vi "HTTP Info.vi"() -> ()   [LabVIEW 2020, in "VectoScratch.lvlib"]
uses:
  VectoScratch.lvlib
  Vecto/Vecto Info.ctl
  Vecto/Connection Info.ctl
  Vecto/Connection Type.ctl
  Vecto/proto/Discovery/Data.ctl
  Vecto/proto/Service/Data.ctl
  Vecto/proto/ServiceType/Enumeration.ctl
  Vecto/Node/Node Info.ctl
  Vecto/Discovery Info.ctl
  Vecto/VectoService/VectoService.lvclass
  C:/dev/lv20CE/lv-vecto/Vecto/Service/Service.lvclass
  Vecto/DiscoveryService/DiscoveryService.lvclass
  Vecto/Node/Node.lvclass
  Vecto/Vecto/Vecto.lvclass
  Vecto/Vecto.lvlib
  Vecto/proto/ServiceType/ServiceType.lvlib
  Vecto/proto/Service/Service.lvlib
  Vecto/proto/Discovery/Discovery.lvlib
panel:
  in  "ID":u32=1
  in  "Start":bool
  out "Discovery":T1[](array[typedef]) {"ip" format="%.0x"}
  in  "Discovery Address":string="230.0.0.50"
  in  "Discovery Port":u16=36986
  out "error out":errorcluster
  out "Vecto Info":T4
  in  "stop":bool
  in  "Node Name":string="Alpha"
  in  "HTTP Port":u16=36987
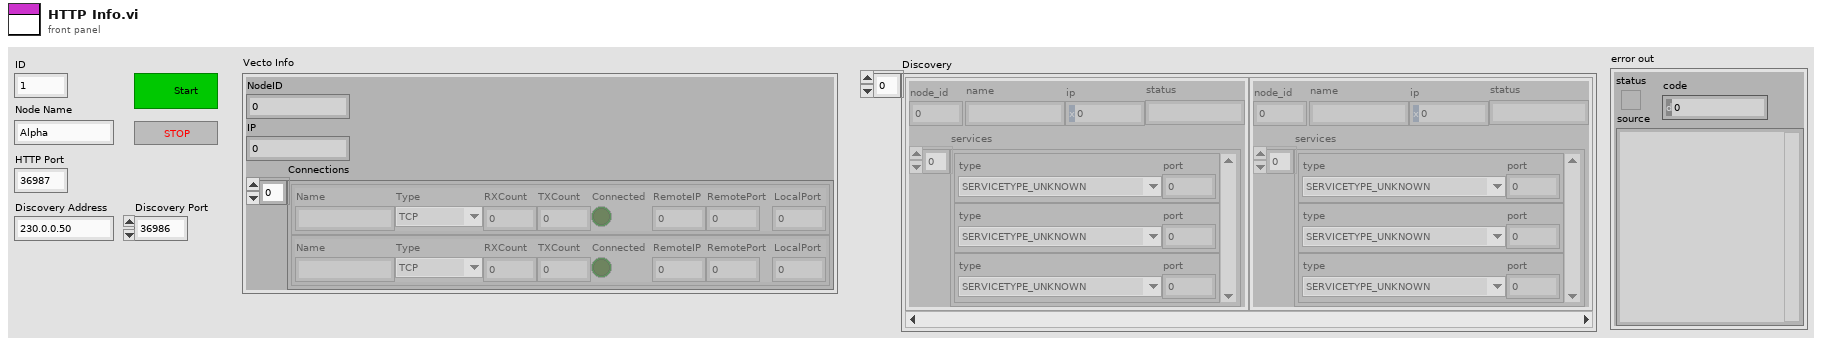
[diagram p1: front panel]
types:
  T1 = typedef "Discovery.lvlib/Data.ctl" = cluster{"node_id":u32, "name":string, "ip":u32, "status":string, "services":T2[]}
  T2 = typedef "Service.lvlib/Data.ctl" = cluster{"type":T3, "port":i32}
  T3 = typedef "ServiceType.lvlib/Enumeration.ctl" = enum16{"SERVICETYPE_UNKNOWN", "SERVICETYPE_TCPSERVER", "SERVICETYPE_HTTPSERVER"}
  T4 = typedef "Vecto.lvlib/Vecto Info.ctl" = cluster{"NodeID":i32, "IP":u32, "Connections":T5[]}
  T5 = typedef "Vecto.lvlib/Connection Info.ctl" = cluster{"Name":string, "Type":T6, "RXCount":i32, "TXCount":i32, "Connected":bool, "RemoteIP":u32, "RemotePort":u16, "LocalPort":u16}
  T6 = typedef "Vecto.lvlib/Connection Type.ctl" = enum16{"TCP", "Telemetry", "Discovery", "HTTP"}
  T7 = typedef "Vecto.lvlib/Discovery Info.ctl" = cluster{"Address":string, "Port":u16, "Interval S":dbl}
  T8 = typedef "Vecto.lvlib/Node.lvclass/Node Info.ctl" = cluster{"HTTP Port":u16, "Bind Address":string}
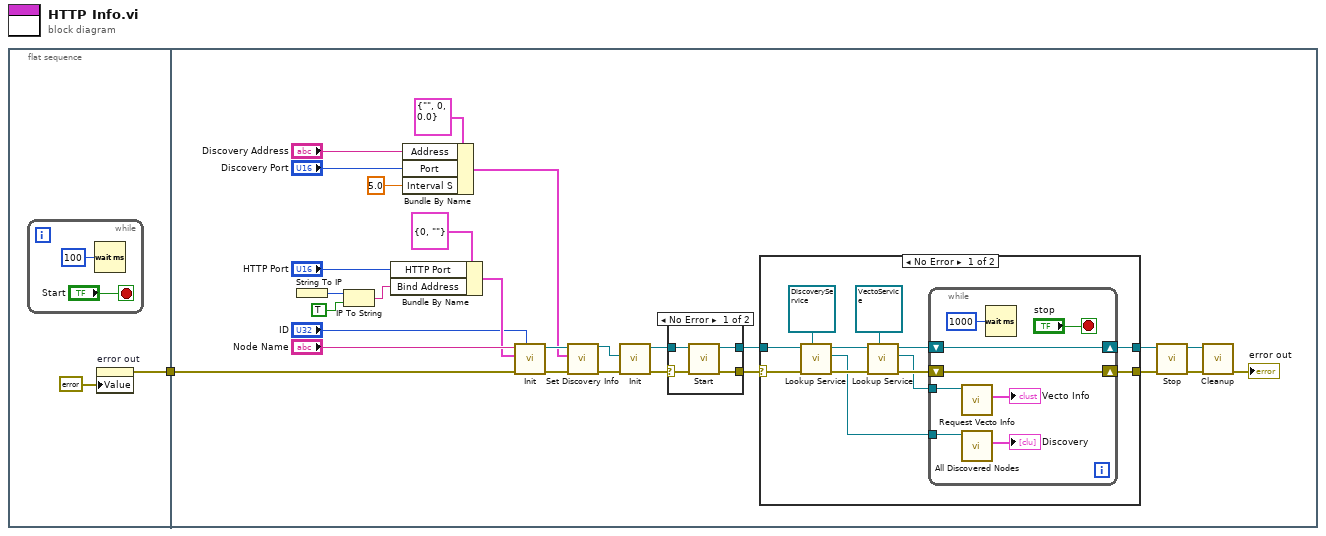
[diagram p0: block diagram]
diagram:
  n1 = flat-sequence {
    tunnel: [w2] -> w1
    tunnel: w1 -> [w7]
    frame #0 {
      n2 = while {
        stop <- "Start" stop-if-true
        n3 = Wait (ms)(milliseconds to wait=u32 100) -> ()  [unwired: 1 out]
      }
      n4 = property on="error out" class="Clust (strict)"("Value"=errorcluster {"status"=FALSE, "code"=0, "source"=""} ("error constant")) -> (error out=w2:errorcluster)  [unwired: 2 in, 1 out]
    }
    frame #1 {
      n5 = String To IP() -> (0:w17:u32)  [unwired: 1 in]
      n6 = IP To String(1:TRUE ("dot notation? (F)"), 2:w17) -> (0:w18:string)
      n7 = Bundle By Name(cluster=T8 {"HTTP Port"=0, "Bind Address"=""} ("Node Info"), "HTTP Port"="HTTP Port", "Bind Address"=w18) -> (w8:T8)
      n8 = Bundle By Name(cluster=T7 {"Address"="", "Port"=0, "Interval S"=0.0} ("Discovery Info"), "Address"="Discovery Address", "Port"="Discovery Port", "Interval S"=5.0) -> (w12:T7)
      n9 = call "Init.vi"("ID"="ID", "error in (no error)"=w7, "Node Info"=w8, "Name"="Node Name") -> ("error out"=w29:errorcluster, "Node out"=w15:refnum<class "Node.lvclass">)  [unwired: 6 in]
      n10 = call "Set Discovery Info.vi"("error in (no error)"=w29, "Discovery Info"=w12, "Node in"=w15) -> ("error out"=w16:errorcluster, "Node out"=w14:refnum<class "Node.lvclass">)  [unwired: 7 in]
      n11 = call "Init.vi"("error in (no error)"=w16, "Node"=w14) -> ("error out"=w28:errorcluster, "Vecto out"=w27:refnum<class "Vecto.lvclass">)  [unwired: 8 in]
      n12 = case shown="No Error" w28 {
        selector: w28 -> [w36 w38]
        tunnel: w27 -> [w35 w37]
        tunnel: [w34 w38] -> w26
        tunnel: [w33 w37] -> w23
        frame No Error {
          n13 = call "Start.vi"("error in (no error)"=w36, "Vecto in"=w35) -> ("error out"=w34:errorcluster, "Vecto out"=w33:refnum<class "Vecto.lvclass">)  [unwired: 8 in]
        }
        frame Error {
        }
      }
      n14 = case shown="No Error" w26 {
        selector: w26 -> [w43 w60]
        tunnel: [w50 w59] -> w25
        tunnel: [w49 w60] -> w24
        tunnel: w23 -> [w44 w59]
        frame No Error {
          n15 = call "Lookup Service.vi"("Service Type / ID"=refnum<class "DiscoveryService.lvclass"> refnum ("Vecto.lvlib:DiscoveryService.lvclass"), "error in (no error)"=w43, "Vecto in"=w44) -> ("error out"=w42:errorcluster, "Service"=w39:refnum<class "DiscoveryService.lvclass">, "Vecto out"=w41:refnum<class "Vecto.lvclass">)  [unwired: 6 in]
          n16 = call "Lookup Service.vi"("Service Type / ID"=refnum<class "VectoService.lvclass"> refnum ("Vecto.lvlib:VectoService.lvclass"), "error in (no error)"=w42, "Vecto in"=w41) -> ("error out"=w48:errorcluster, "Service"=w45:refnum<class "VectoService.lvclass">, "Vecto out"=w47:refnum<class "Vecto.lvclass">)  [unwired: 6 in]
          n17 = while {
            shift-right: [w56] -> w49
            shift-left: w48 -> [w56]
            shift-right: [w57] -> w50
            shift-left: w47 -> [w57]
            tunnel: w45 -> [w54]
            tunnel: w39 -> [w52]
            stop <- "stop" stop-if-true
            n18 = call "Request Vecto Info.vi"("VectoService in"=w54) -> ("Vecto Info"=→"Vecto Info":T4)  [unwired: 8 in, 2 out]
            n19 = call "All Discovered Nodes.vi"("DiscoveryService in"=w52) -> ("Nodes"=→"Discovery":T1[])  [unwired: 8 in, 2 out]
            n20 = Wait (ms)(milliseconds to wait=u32 1000) -> ()  [unwired: 1 out]
          }
        }
        frame Error {
        }
      }
      n21 = call "Stop.vi"("error in (no error)"=w24, "Vecto in"=w25) -> ("error out"=w22:errorcluster, "Vecto out"=w21:refnum<class "Vecto.lvclass">)  [unwired: 8 in]
      n22 = call "Cleanup.vi"("error in (no error)"=w22, "Vecto in"=w21) -> ("error out"=→"error out":errorcluster)  [unwired: 9 in]
    }
  }
